vi "Teardown.vi"(8 "error in (no error)":errorcluster, 11 "LUnit Test Max File Size (SQL) In":refnum<class "Test Max File Size (SQL).lvclass">) -> (0 "error out":errorcluster, 3 "LUnit Test Max File Size (SQL) Out":refnum<class "Test Max File Size (SQL).lvclass">)   [LabVIEW 2019, in "Test Max File Size (SQL).lvclass"]
doc: "Teardown method called by the testing framework to tear down test fixture after each test method is called."
uses:
  Test Max File Size (SQL).lvclass
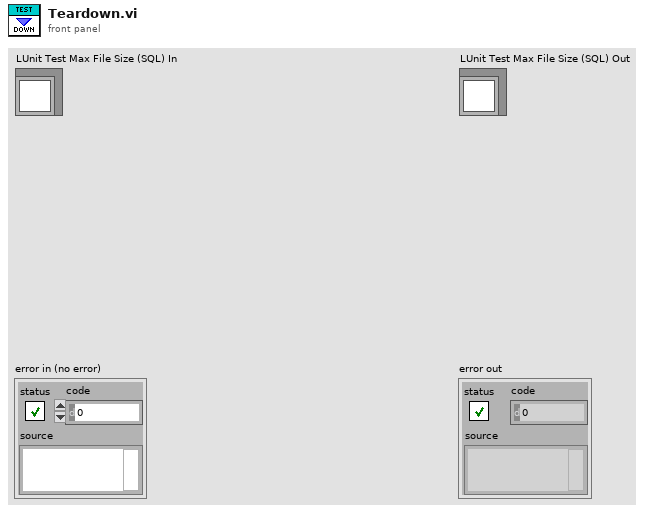
[diagram p1: front panel]
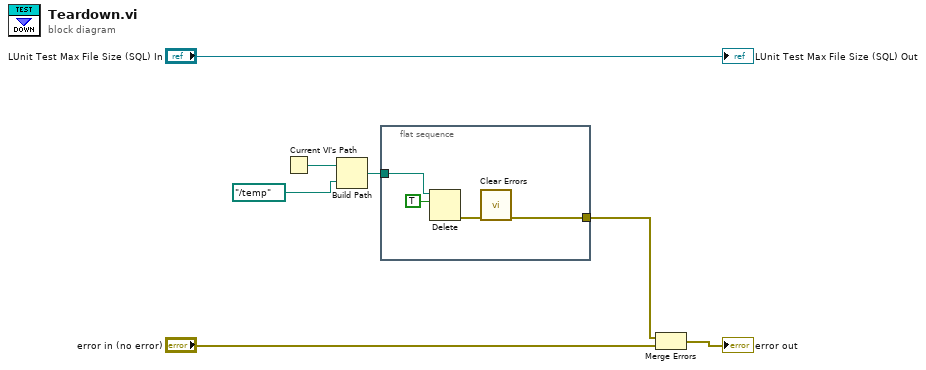
[diagram p0: block diagram]
diagram:
  n1 = Current VI's Path() -> (path=w5:path)
  n2 = Build Path(base path=w5, name or relative path=path "../temp") -> (appended path=w3:path)
  n3 = flat-sequence {
    tunnel: w3 -> [w11]
    tunnel: [w8] -> w1
    frame #0 {
      n4 = Delete(path (use dialog)=w11, entire hierarchy (F)=TRUE) -> (error out=w10:errorcluster)  [unwired: 3 in, 2 out]
      n5 = call <vilib>:"Clear Errors.vi"("error in (no error)"=w10) -> ("error out"=w8:errorcluster)  [unwired: 5 in, 1 out]
    }
  }
  n6 = Merge Errors(w1, "error in (no error)") -> (→"error out":errorcluster)
  "LUnit Test Max File Size (SQL) Out" <- "LUnit Test Max File Size (SQL) In"
